vi "InitString.vi"(8 "ErrorArray in":errorcluster[](array[cluster]), 10 "StringRefArray":refnum<vi>[](array[refnum]), 11 "IniFileRef in":T1) -> (0 "ErrorArray Out":errorcluster[](array[cluster]), 3 "IniFileRef out":T1)   [LabVIEW 2014, in "Ini_lib.lvlib"]
uses:
  Ini_lib.lvlib
  <vilib>/Utility/config.llb/Config Data RefNum.ctl
  <userlib>/NIST/NISTErrorLib/NISTErrorLib.lvlib
  <vilib>/Utility/config.llb/NI_LVConfig.lvlib
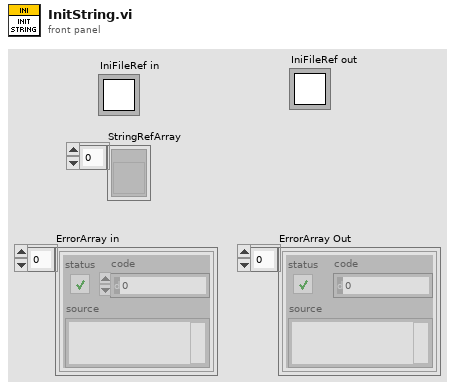
[diagram p1: front panel]
types:
  T1 = typedef "NI_LVConfig.lvlib/Config Data RefNum.ctl" = refnum<k1>
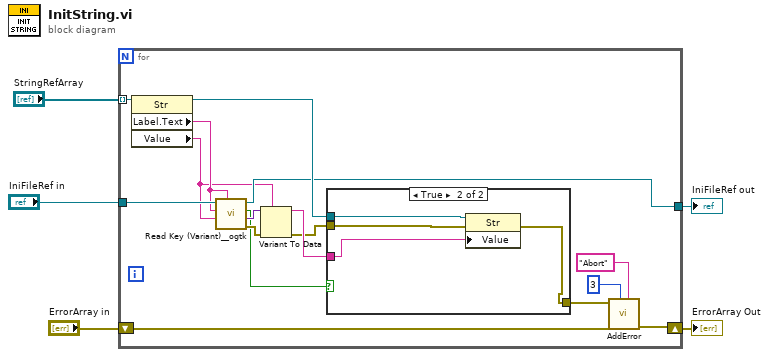
[diagram p0: block diagram]
diagram:
  n1 = for {
    tunnel: "StringRefArray" -> [w17] mode=indexing
    tunnel: "IniFileRef in" -> [w19]
    tunnel: [w14] -> w5
    shift-right: [w12] -> w1
    shift-left: "ErrorArray in" -> [w13]
    n2 = property class="Str"(reference=w17) -> (reference out=w16:refnum<vi>, "Label.Text"=w7:string, "Value"=w6:string)  [unwired: 1 in, 1 out]
    n3 = call <userlib>:"Read Key (Variant)__ogtk.vi"("section"=w7, "type"=w6, "key (optional)"=w7, "refnum"=w19) -> ("error out"=w21:errorcluster, "key-value"=w20:variant, "found?"=w8:bool, "refnum out"=w14:T1)  [unwired: 4 in]
    n4 = Variant To Data(error in=w21, type=w6, Variant=w20) -> (data=w18:string, error out=w15:errorcluster)
    n5 = case shown="True" w8 {
      tunnel: w18 -> [_ w23]
      tunnel: w16 -> [_ w26]
      tunnel: w15 -> [w22 w25]
      tunnel: [w22 w24] -> w11
      frame False {
      }
      frame True {
        n6 = property class="Str"(reference=w26, error in=w25, "Value"=w23) -> (error out=w24:errorcluster)  [unwired: 1 out]
      }
    }
    n7 = call <userlib>:"AddError.vi"("Severity"="Abort", "Priority"=u8 3, "ErrorArray"=w13, "error in (no error)"=w11) -> ("ErrorArray"=w12:errorcluster[])  [unwired: 6 in, 1 out]
  }
  "ErrorArray Out" <- w1
  "IniFileRef out" <- w5
